vi "ShowPanel.vi"(8 "error in (no error)":errorcluster, 11 "Task_Abstr in":refnum<class "Task_Abstr.lvclass">) -> (0 "error out":errorcluster, 2 "FP.NativeWindow":u64, 3 "Task_Abstr out":refnum<class "Task_Abstr.lvclass">)   [LabVIEW 2025, in "Task_Abstr.lvlib" / "Task_Abstr.lvclass"]
uses:
  Task_Abstr.lvclass
  Task_Abstr.lvclass/Task_Abstr.ctl
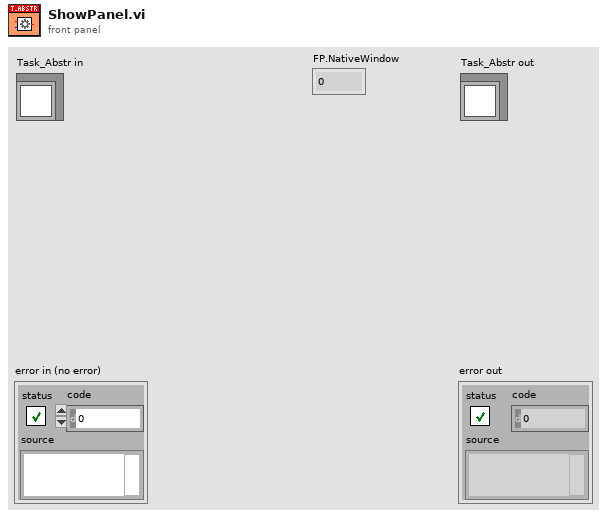
[diagram p1: front panel]
types:
  T1 = enum32{"Invalid", "Standard", "Closed", "Hidden", "Minimized", "Maximized"}
  T2 = typedef "DAQ_Module.lvlib/DAQ_Module.lvclass/DAQ_Task_Config.ctl" = cluster{"Drive":T3, "TaskType":T4, "PhysicalChannels":string, "SampleRateConfiguration":T5, "ChannelConfig":string, "Enable":bool}
  T3 = typedef "DAQ_Module.lvlib/DAQ_Module.lvclass/DAQ_HW_Type.ctl" = enum16{"NI_DAQmx", "Simulated_DAQ"}
  T4 = typedef "DAQ_Module.lvlib/DAQ_Module.lvclass/DAQ_Task_Type.ctl" = enum16{"AI", "Linear", "Angular", "AO"}
  T5 = typedef "DAQ_Module.lvlib/DAQ_Module.lvclass/DAQ_SampleRateConfig.ctl" = cluster{"SampleRate":dbl, "SamplesPerChannel":u32, "SamplesPerRead":i32, "SampleMode":i32, "Clock Source":string}
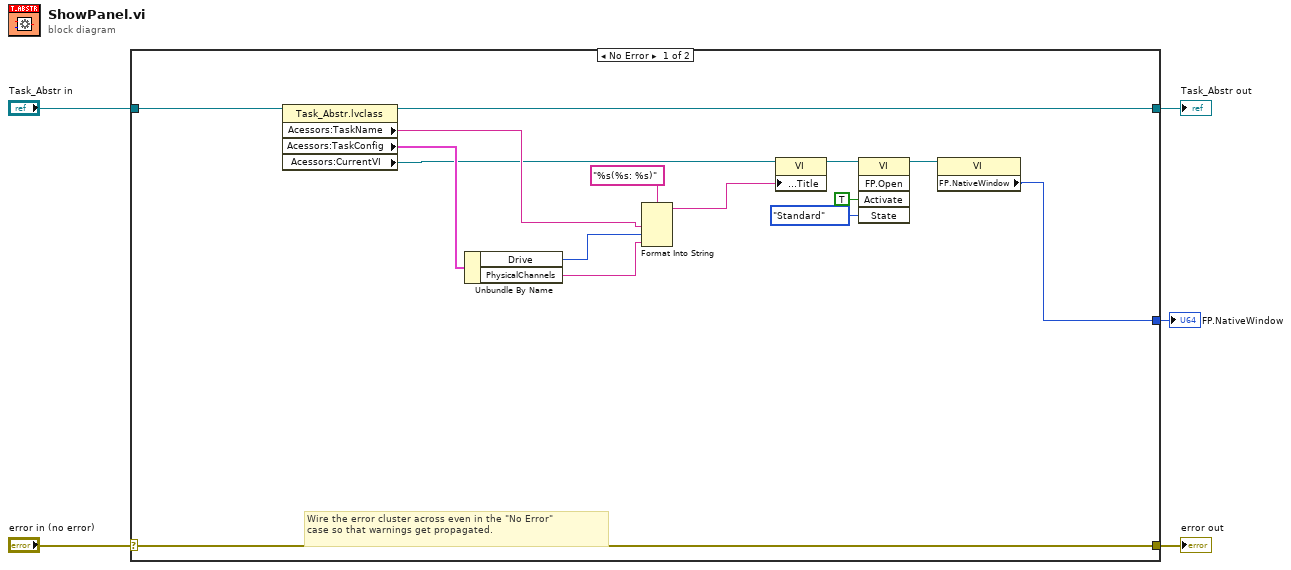
[diagram p0: block diagram]
diagram:
  n1 = case shown="No Error" "error in (no error)" {
    selector: "error in (no error)" -> [w20 w22]
    tunnel: [w20 w22] -> w4
    tunnel: [w13 w21] -> w2
    tunnel: "Task_Abstr in" -> [w14 w21]
    tunnel: [w6 _] -> w1
    frame No Error {
      # "Wire the error cluster across even in the \"No Error\"\ncase so that warnings get propagated."
      n2 = property class="Task_Abstr.lvclass"(reference=w14) -> (reference out=w13:refnum<class "Task_Abstr.lvclass">, "Acessors:TaskName"=w12:string, "Acessors:TaskConfig"=w16:T2, "Acessors:CurrentVI"=w11:refnum<vi>)  [unwired: 1 in, 1 out]
      n3 = Unbundle By Name(w16) -> ("Drive"=w9:T3, "PhysicalChannels"=w8:string)
      n4 = Format Into String(format string="%s(%s: %s)", w12, w9, w8) -> (resulting string=w15:string)  [unwired: 2 in, 1 out]
      n5 = property class="VI"(reference=w11, "Front Panel.Title"=w15) -> (reference out=w19:refnum<vi>)  [unwired: 1 in, 1 out]
      n6 = invoke class="VI" method="FP.Open"(reference=w19, "Activate"=TRUE ("Activate?"), "State"=T1."Standard") -> (reference out=w7:refnum<vi>)  [unwired: 2 in, 4 out]
      n7 = property class="VI"(reference=w7) -> ("FP.NativeWindow"=w6:u64)  [unwired: 1 in, 2 out]
    }
    frame Error {
    }
  }
  "error out" <- w4
  "Task_Abstr out" <- w2
  "FP.NativeWindow" <- w1
